vi "oa_FIR Preprocess Filter Error Handler (Multiple).vi"(8 "error in (no error)":errorcluster, 9 "condition failed?":bool[](array[boolean]), 10 "error sources":i32[](array[numeric])) -> (0 "error out":errorcluster)   [LabVIEW 2017, in "SoundVib_RefDataProcess.lvlib"]
uses:
  <vilib>/addons/Sound and Vibration/Order Analysis/Referece Data Processing/SoundVib_RefDataProcess.lvlib
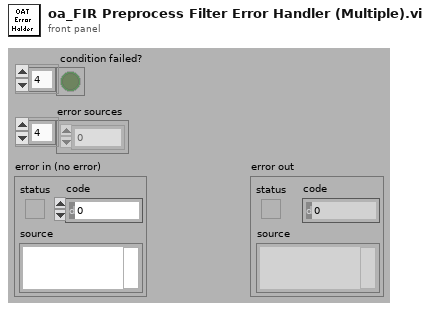
[diagram p1: front panel]
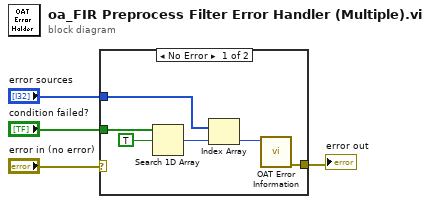
[diagram p0: block diagram]
diagram:
  n1 = case shown="No Error" "error in (no error)" {
    selector: "error in (no error)" -> [_ w11]
    tunnel: [w5 w11] -> w3
    tunnel: "condition failed?" -> [w8 _]
    tunnel: "error sources" -> [w7 _]
    frame No Error {
      n2 = Search 1D Array(1D array=w8, element=TRUE) -> (index of element=w9:i32)  [unwired: 1 in]
      n3 = Index Array(array=w7, index=w9) -> (element=w6:i32)
      n4 = call <vilib>:"OAT Error Information.vi"("error code"=w6) -> ("error out"=w5:errorcluster)  [unwired: 6 in]
    }
    frame Error {
    }
  }
  "error out" <- w3
